vi "onCheckConnection.vi"(8 "error in (no error)":errorcluster, 11 "Connection in":refnum<class "Connection.lvclass">) -> (0 "error out":errorcluster, 2 "connection OK":bool, 3 "Connection out":refnum<class "Connection.lvclass">)   [LabVIEW 2013, in "Connection_GOSPL.lvlib" / "Connection.lvclass"]
uses:
  Connection.lvclass
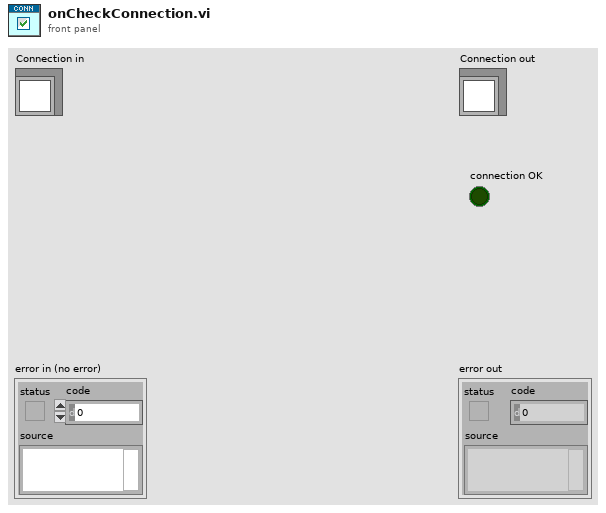
[diagram p1: front panel]
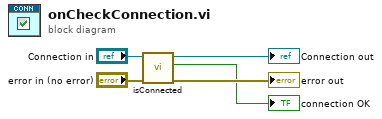
[diagram p0: block diagram]
diagram:
  n1 = call "isConnected.vi"("error in (no error)"="error in (no error)", "Connection in"="Connection in") -> ("error out"=→"error out":errorcluster, "connected"=→"connection OK":bool, "Connection out"=→"Connection out":refnum<class "Connection.lvclass">)  [unwired: 7 in]
